vi "Mulit String to one row string.vi"(8 "error in (no error)":errorcluster, 11 "XML String":string) -> (0 "error out":errorcluster, 2 "Final size(s)":i32, 3 "one row string":string, 5 "Array":string[](array[string]))   [LabVIEW 2021]
doc: "multi row string to one row string"
panel:
  out "Original array":string[](array[string])
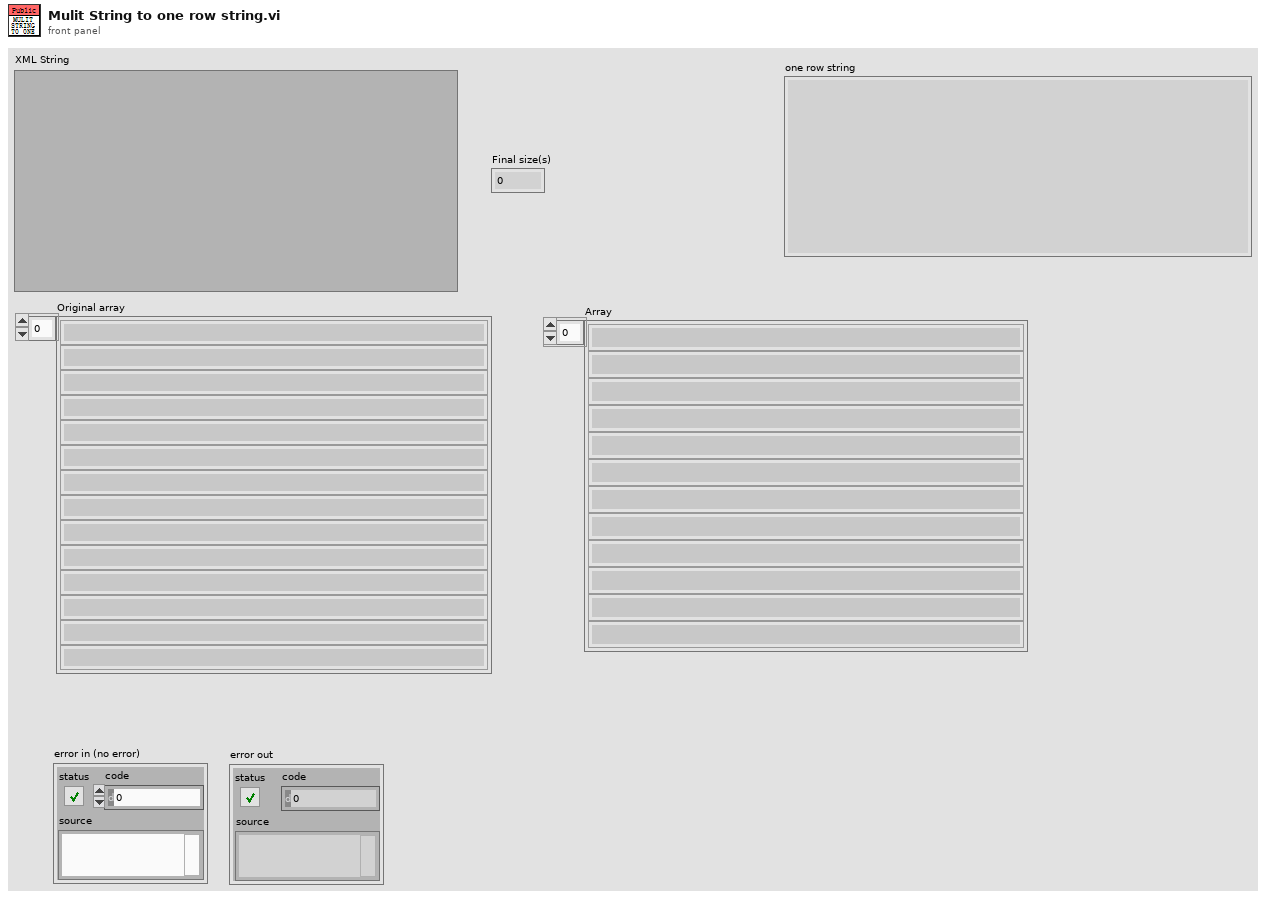
[diagram p1: front panel]
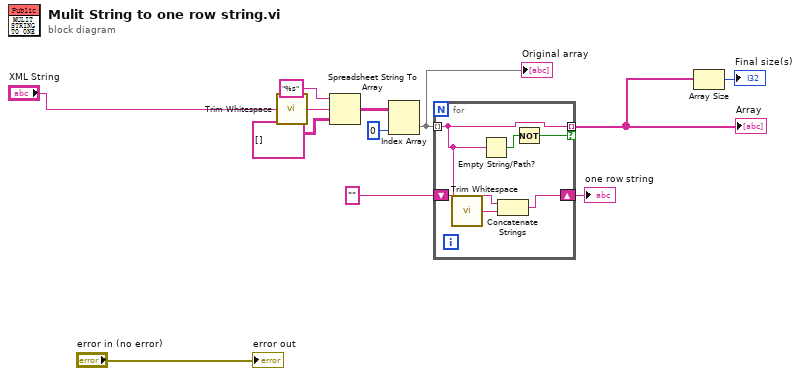
[diagram p0: block diagram]
diagram:
  n1 = call <vilib>:"Trim Whitespace.vi"("string"="XML String") -> ("trimmed string"=w3:string)  [unwired: 1 in]
  n2 = Spreadsheet String To Array(format string="%s", spreadsheet string=w3, array type (2D Dbl)=string[][] []) -> (array=w6:string[][])  [unwired: 1 in]
  n3 = Index Array(array=w6, index (col)=0 ("disabled index (col)")) -> (element=w4:string[])  [unwired: 1 in]
  "Original array" <- w4
  n4 = for {
    tunnel: w4 -> [w16] mode=indexing
    tunnel: [w16] -> w9 mode=indexing if=w17
    shift-right: [w14] -> w12
    shift-left: "" ("format string") -> [w15]
    n5 = call <vilib>:"Trim Whitespace.vi"("string"=w16) -> ("trimmed string"=w13:string)  [unwired: 1 in]
    n6 = Empty String/Path?(string/path=w16) -> (empty?=w18:bool)
    n7 = Concatenate Strings(w15, w13) -> (w14:string)
    n8 = Not(x=w18) -> (.not. x?=w17:bool)
  }
  "Array" <- w9
  "one row string" <- w12
  n9 = Array Size(array=w9) -> (size(s)=→"Final size(s)":i32)
  "error out" <- "error in (no error)"
